vi "Load Constants if robot is first call or dashboard commands it.vi"(8 "error in (no error)":errorcluster) -> (0 "error out":errorcluster)   [LabVIEW 2013]
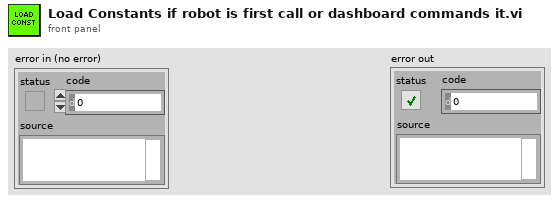
[diagram p1: front panel]
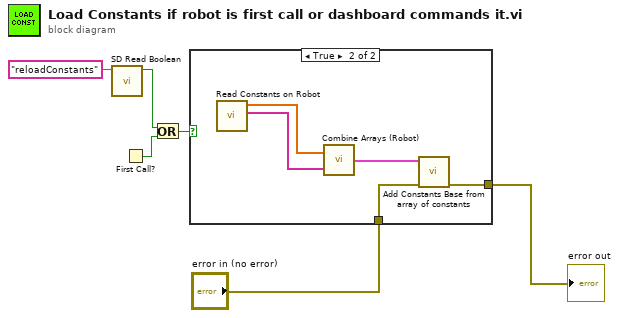
[diagram p0: block diagram]
diagram:
  n1 = call <vilib>:"SD Read Boolean.vi"("Name"="reloadConstants") -> ("Boolean"=w5:bool)  [unwired: 8 in, 2 out]
  n2 = First Call?() -> (First Call?: T/F=w4:bool)
  n3 = Or(x=w5, y=w4) -> (x .or. y?=w3:bool)
  n4 = case shown="True" w3 {
    tunnel: "error in (no error)" -> [w7 w9]
    tunnel: [w7 w8] -> w1
    frame False {
    }
    frame True {
      n5 = call "Read Constants on Robot.vi"() -> ("Constant Names"=w11:string[], "Constant Values"=w12:dbl[])  [unwired: 10 in]
      n6 = call "Combine Arrays (Robot).vi"("Variable Names"=w11, "Array of Numbers"=w12) -> ("Constants"=w10:cluster{"output string":string, dbl}[])
      n7 = call "Add Constants Base from array of constants.vi"("error in (no error)"=w9, "Constants Array"=w10) -> ("error out"=w8:errorcluster)  [unwired: 9 in]
    }
  }
  "error out" <- w1
